vi "test_riccat_04Ni.vi"() -> (3 "All Tests Passed":bool)   [LabVIEW 2019]
uses:
  <vilib>/Rock Robotics/WPI/ThirdParty/JAS_Junk/TrajLib/Trajectory_Library.lvlib
  <vilib>/Analysis/NI_AALPro.lvlib
  <vilib>/Analysis/7linalg.llb/Solve Linear Equations (multiple right hand).vi
  <vilib>/Analysis/7linalg.llb/Real Transpose Matrix.vi
  <vilib>/Analysis/Matrix/Datatypes/RealMatrix.ctl
  <vilib>/Analysis/Matrix/NI_Matrix.lvlib
panel:
  out "error 2":i32
  out "error":i32
  out "Solution Matrix":T1
  out "R1":T1
  out "Q1":T1
  out "N1":T1
  in  "N":T1=[[1.0, 0.0], [0.0, 1.0]]
  out "error out 2":errorcluster
  out "Pos Semi Definite":bool
  out "Q_Chk_Passed":bool
  out "C":T1
  out "Q Check":T1
  out "Bad":bool
  out "Stable Bad":bool
  out "error out":errorcluster
  out "Eigenvalues":cdb[](array[numeric])
  out "Error":bool
  out "Iterations":i32
  out "Elapsed \nTime MS":dbl
  out "ZERO":T1
  out "X  Answer":T1
  in  "R":T1=[[1.0, 0.0], [0.0, 1.0]]
  in  "Q":T1=[[1.0, 0.0], [0.0, 1.0]]
  in  "B":T1=[[1.0, 0.0], [0.0, 1.0]]
  in  "A":T1=[[1.0, 0.0], [0.0, 1.0]]
  # "// ------------------------------------------------------------\n  // Test 4: A = B = Q = R = I_2 (2-by-2 identity matrix)"
  # "A4 << \n           1, 0, \n            0, 1;"
  # "B4 << \n    1, \n    0, \n    0, \n    1;"
  # "Solution weight ??"
  # "Q4 << \n        1, 0, \n         0, 1;"
  # "Cost ??"
  # "R4 << \n        1, 0, \n        0, 1;"
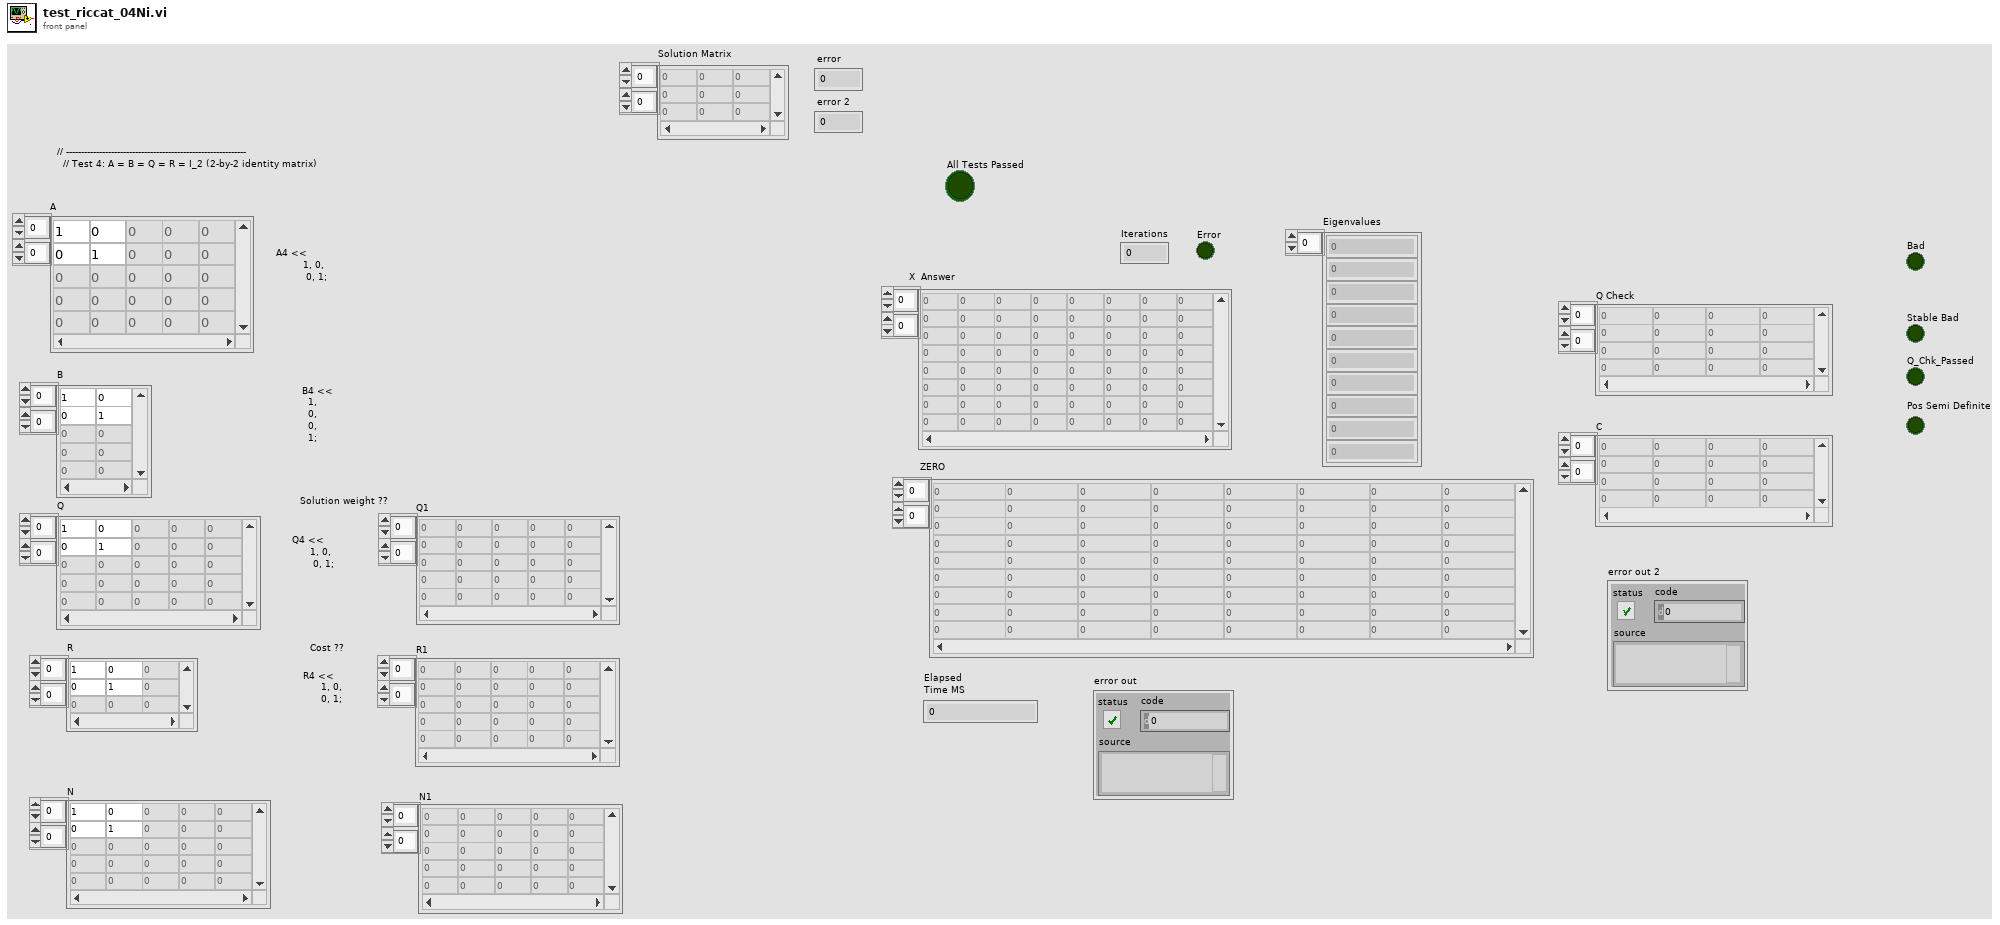
[diagram p1: front panel]
types:
  T1 = typedef "NI_Matrix.lvlib/RealMatrix.ctl" = dbl[][]
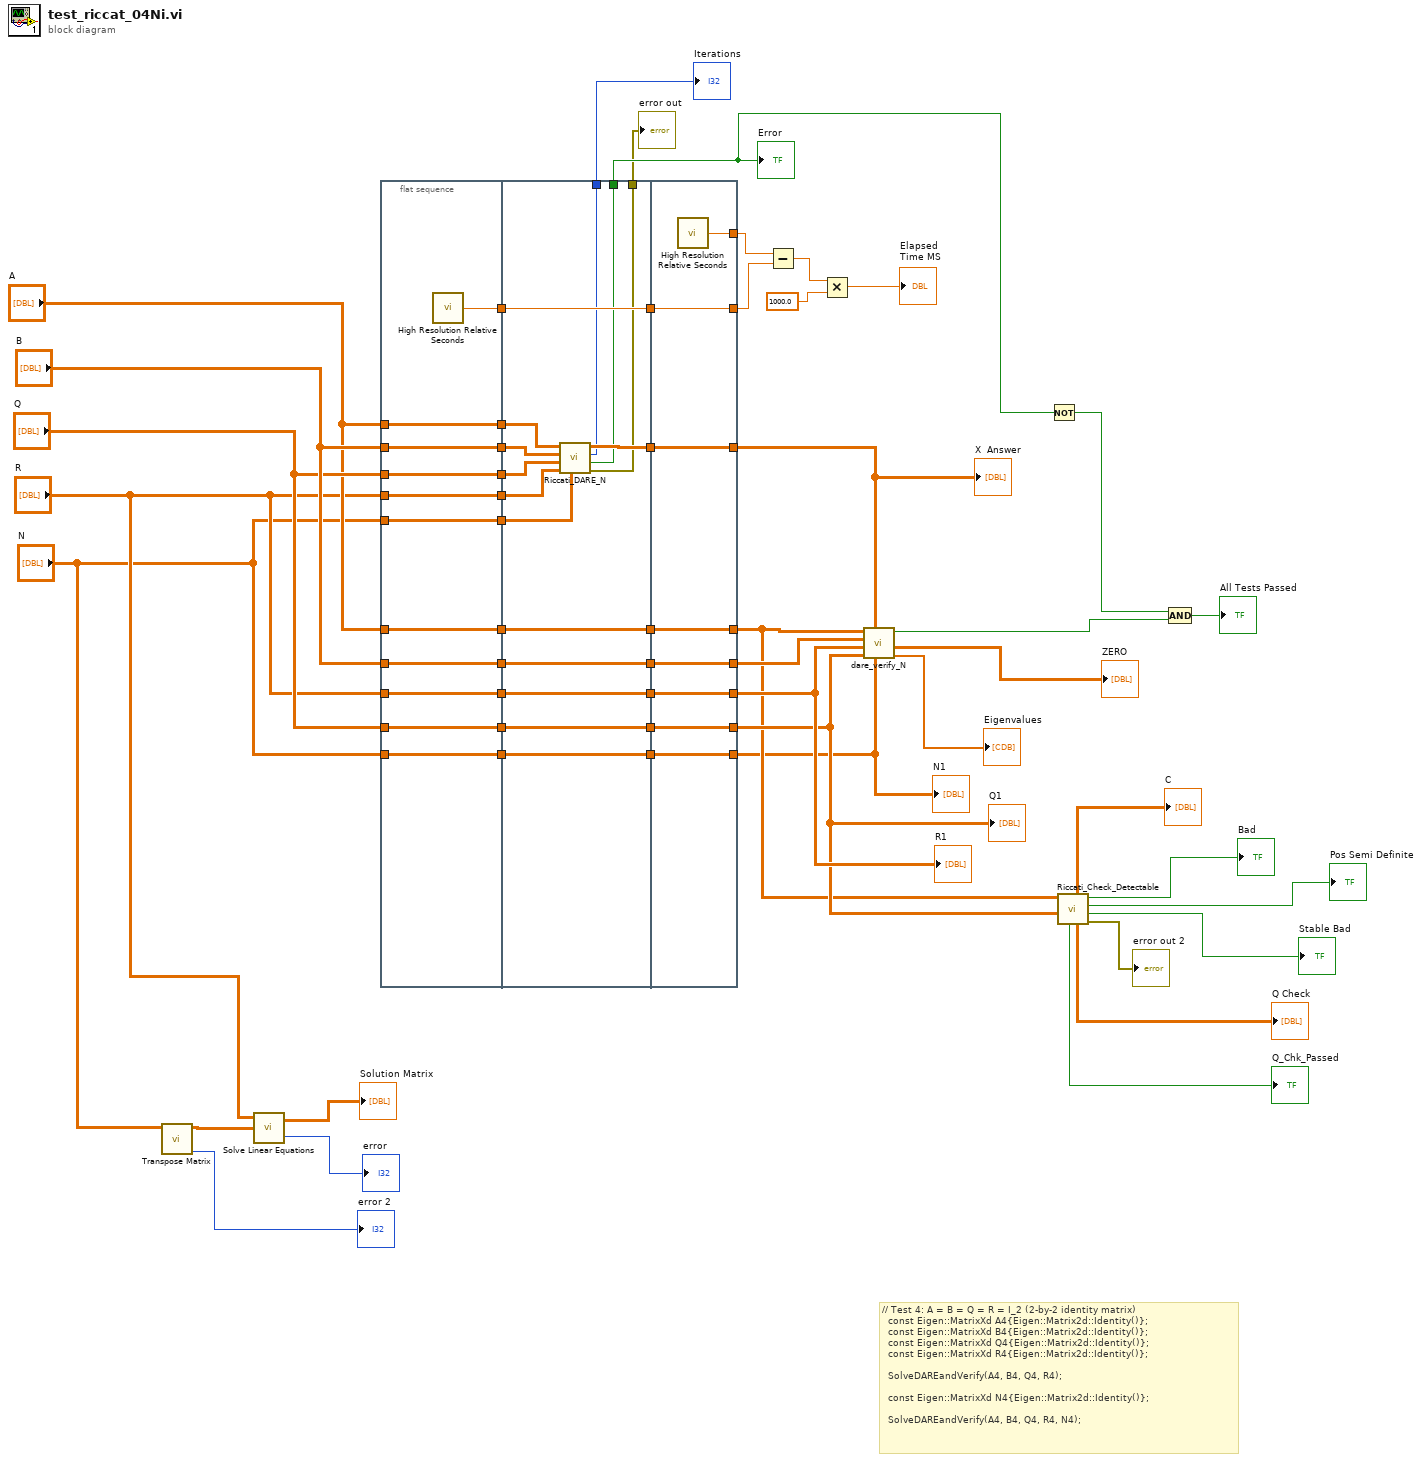
[diagram p0: block diagram]
diagram:
  # "// Test 4: A = B = Q = R = I_2 (2-by-2 identity matrix)\n  const Eigen::MatrixXd A4{Eigen::Matrix2d::Identity()};\n  const Eigen::MatrixXd B4{Eigen::Matrix2d::Identity()};\n  const Eigen::MatrixXd Q4{Eigen::Matrix2d::Identity()};\n  const Eigen::MatrixXd R4{Eigen::Matrix2d::Identity()};\n\n  SolveDAREandVerify(A4, B4, Q4, R4);\n\n  const Eigen::MatrixXd N4{Eigen::Matrix2d::Identity()};\n\n  SolveDAREandVerify(A4, B4, Q4, R4, N4);"
  n1 = call-poly <vilib>:"Transpose Matrix.vi"("Input Matrix"="N") -> ("error"=→"error 2":i32, "Matrix Transpose"=w5:T1)  [unwired: 9 in]
  n2 = call-poly <vilib>:"Solve Linear Equations.vi"("Known Matrix"=w5, "Input Matrix"="R") -> ("error"=→"error":i32, "Solution Matrix"=→"Solution Matrix":T1)  [unwired: 1 in]
  n3 = flat-sequence {
    tunnel: "B" -> [w59]
    tunnel: "A" -> [w60]
    tunnel: "B" -> [w61]
    tunnel: "Q" -> [w62]
    tunnel: "A" -> [w63]
    tunnel: "R" -> [w64]
    tunnel: [w64] -> w53
    tunnel: [w63] -> w52
    tunnel: [w62] -> w51
    tunnel: [w61] -> w50
    tunnel: [w60] -> w49
    tunnel: [w59] -> w48
    tunnel: "R" -> [w58]
    tunnel: [w58] -> w43
    tunnel: "Q" -> [w57]
    tunnel: [w57] -> w42
    tunnel: [w56] -> w37
    tunnel: [w55] -> w12
    tunnel: "N" -> [w55]
    tunnel: "N" -> [w54]
    tunnel: [w54] -> w9
    tunnel: w53 -> [w79]
    tunnel: w52 -> [w77]
    tunnel: w51 -> [w76]
    tunnel: w50 -> [w75]
    tunnel: w49 -> [w74]
    tunnel: w48 -> [w73]
    tunnel: [w78] -> w47
    tunnel: [w74] -> w46
    tunnel: [w73] -> w45
    tunnel: [w72] -> w44
    tunnel: w43 -> [w72]
    tunnel: w42 -> [w71]
    tunnel: [w71] -> w41
    tunnel: [w70] -> w38
    tunnel: w37 -> [w70]
    tunnel: [w69] -> w33
    tunnel: [w68] -> w32
    tunnel: [w67] -> w24
    tunnel: w12 -> [w66]
    tunnel: [w65] -> w10
    tunnel: w9 -> [w65]
    tunnel: [w85] -> w20
    tunnel: [w86] -> w18
    tunnel: [w87] -> w31
    tunnel: w47 -> [w87]
    tunnel: w46 -> [w86]
    tunnel: w45 -> [w85]
    tunnel: [w84] -> w30
    tunnel: w44 -> [w84]
    tunnel: w41 -> [w81]
    tunnel: [w83] -> w40
    tunnel: [w82] -> w39
    tunnel: w38 -> [w82]
    tunnel: [w81] -> w19
    tunnel: [w80] -> w11
    tunnel: w10 -> [w80]
    frame #0 {
      n4 = call <vilib>:"High Resolution Relative Seconds.vi"() -> ("relative seconds"=w56:dbl)
    }
    frame #1 {
      n5 = call <vilib>:"Riccati_DARE_N.vi"("N"=w66, "R"=w79, "Q"=w76, "B"=w75, "A"=w77) -> ("error out"=w67:errorcluster, "Error"=w68:bool, "Iterations"=w69:i32, "Answer"=w78:T1)  [unwired: 3 in]
    }
    frame #2 {
      n6 = call <vilib>:"High Resolution Relative Seconds.vi"() -> ("relative seconds"=w83:dbl)
    }
  }
  n7 = Subtract(x=w40, y=w39) -> (x-y=w36:dbl)
  n8 = Multiply(x=w36, y=1000.0) -> (x*y=→"Elapsed \nTime MS":dbl)
  n9 = call "dare_verify_N.vi"("N"=w11, "Answer"=w31, "Q"=w19, "R"=w30, "B"=w20, "A"=w18) -> ("Eigenvalues"=→"Eigenvalues":cdb[], "ZERO"=→"ZERO":T1, "Passed"=w27:bool)  [unwired: 3 in]
  n10 = Not(x=w32) -> (.not. x?=w28:bool)
  n11 = call <vilib>:"Riccati_Check_Detectable.vi"("Q"=w19, "A"=w18) -> ("error out"=→"error out 2":errorcluster, "Stable Bad"=→"Stable Bad":bool, "Pos Semi Definite"=→"Pos Semi Definite":bool, "Bad"=→"Bad":bool, "Q_Check"=→"Q Check":T1, "C"=→"C":T1, "Q_Chk_Passed"=→"Q_Chk_Passed":bool)  [unwired: 3 in]
  n12 = Compound Arithmetic op=AND(w28, w27) -> (→"All Tests Passed":bool)
  "X  Answer" <- w31
  "Iterations" <- w33
  "Error" <- w32
  "error out" <- w24
  "N1" <- w11
  "Q1" <- w19
  "R1" <- w30
